vi "ex_HeaderToSprdsheetStr.vi"(6 "project":string, 7 "operator name":string, 8 "error in (no error)":errorcluster, 9 "Relative Time?":bool, 10 "file params in":T1={"delimiter"="\t", "origin time"=timestamp(0 s since 1904-01-01), "Flags"={"include col headings?"=TRUE, "x_columns"=0, "col headings always?"=TRUE, "time preference"=0, "hide col headings"=FALSE}, "Decimal Separator"=""} {"Flags"."time preference" items=["Absolute", "Relative"]; "Flags"."x_columns" items=["None", "One", "Multiple"]; "origin time" format="%<%X\n%x>T"}, 11 "description":string) -> (0 "error out":errorcluster, 1 "rows":i32, 2 "spreadsheet array":string[][](array[string]), 3 "spreadsheet string":string)   [LabVIEW 2020]
uses:
  <vilib>/express/express output/ExFileWriteBlock.llb/ex_WriteFileParams.ctl
  <vilib>/express/express input/ExFileReadBlock.llb/ex_ReadFileParams.ctl
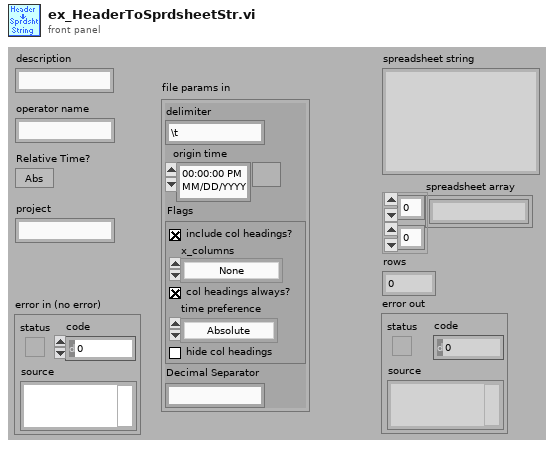
[diagram p1: front panel]
types:
  T1 = typedef "ex_WriteFileParams.ctl" = cluster{"delimiter":string, "origin time":timestamp, "Flags":T2, "Decimal Separator":string}
  T2 = typedef "ex_ReadFileParams.ctl" = cluster{"include col headings?":bool, "x_columns":u16, "col headings always?":bool, "time preference":u16, "hide col headings":bool}
  T3 = typedef "ex_SoftwareRevision.ctl" = cluster{"Major Version":u16, "Minor Version":u16}
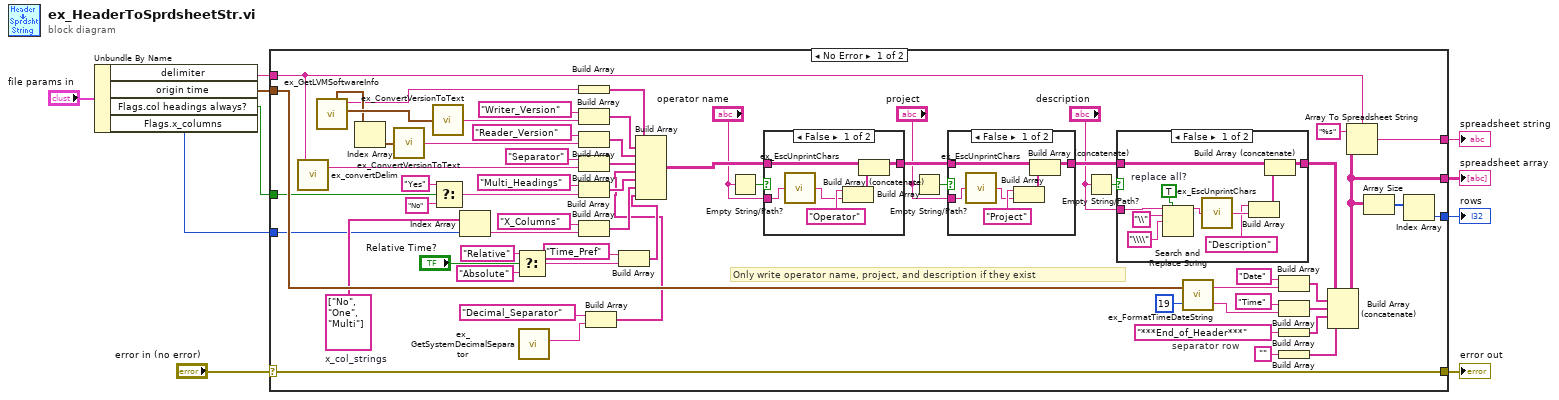
[diagram p0: block diagram]
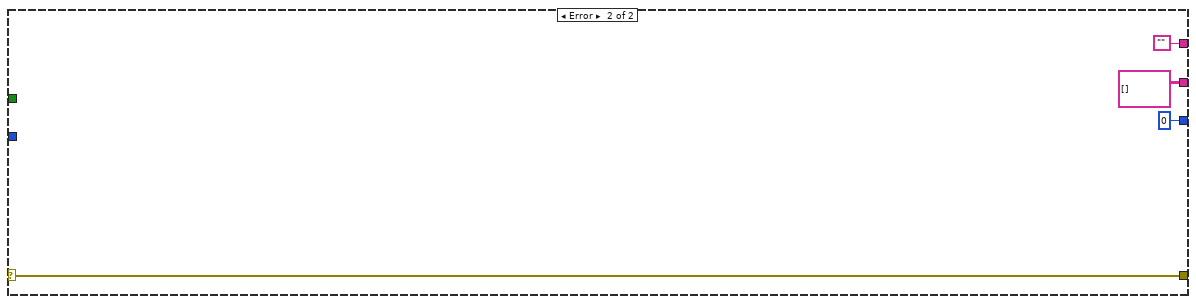
[diagram p5: hidden frame]
diagram:
  n1 = Unbundle By Name("file params in") -> ("delimiter"=w7:string, "origin time"=w6:timestamp, "Flags.col headings always?"=w5:bool, "Flags.x_columns"=w4:u16)
  n2 = case shown="No Error" "error in (no error)" {
    selector: "error in (no error)" -> [w63 w102]
    tunnel: [w63 w102] -> w9
    tunnel: w7 -> [w50 _]
    tunnel: w6 -> [w58 _]
    tunnel: w5 -> [w57 _]
    tunnel: w4 -> [w41 _]
    tunnel: [w20 ""] -> w3
    tunnel: [w19 string[][] []] -> w2
    tunnel: [w18 0] -> w1
    frame No Error {
      w42 = string[] ["No", "One", "Multi"]  # x_col_strings
      # "Only write operator name, project, and description if they exist"
      # "separator row"
      n3 = call <vilib>:"ex_convertDelim.vi"("delimiter in"=w50) -> ("delimiter out"=w51:string)  [unwired: 1 in, 1 out]
      n4 = call <vilib>:"ex_GetLVMSoftwareInfo.vi"() -> ("Version"=w39:T3, "Title"=w34:string, "Write Capabilities"=w37:T3[])  [unwired: 9 out]
      n5 = Index Array(array=w37) -> (element=w35:T3)  [unwired: 1 in]
      n6 = call <vilib>:"ex_ConvertVersionToText.vi"("Version"=w35) -> ("Text Version"=w36:string)
      n7 = call <vilib>:"ex_ConvertVersionToText.vi"("Version"=w39) -> ("Text Version"=w38:string)
      n8 = Select(t="Yes" ("hdr_str_yes"), s=w57, f="No" ("hdr_str_no")) -> (s? t:f=w67:string)
      n9 = Index Array(array=w42, index=w41) -> (element=w40:string)
      n10 = Select(t="Relative" ("hdr_str_yes"), s="Relative Time?", f="Absolute" ("hdr_str_yes")) -> (s? t:f=w49:string)
      n11 = call <vilib>:"ex_GetSystemDecimalSeparator.vi"() -> ("Decimal Seperator"=w11:string)  [unwired: 11 out]
      n12 = Build Array(w34) -> (w56:string[])
      n13 = Build Array("Writer_Version" ("element"), w38) -> (w53:string[])
      n14 = Build Array("Reader_Version" ("element"), w36) -> (w52:string[])
      n15 = Build Array("Separator", w51) -> (w72:string[])
      n16 = Build Array("Multi_Headings" ("hdr_str_rptcolhdgs"), w67) -> (w14:string[])
      n17 = Build Array("X_Columns" ("hdr_str_multtimecol"), w40) -> (w15:string[])
      n18 = Build Array("Decimal_Separator", w11) -> (w12:string[])
      n19 = Build Array("Time_Pref" ("hdr_str_rptcolhdgs"), w49) -> (w16:string[])
      n20 = Build Array(w56, w53, w52, w72, w12, w14, w15, w16) -> (w62:string[][])
      n21 = Empty String/Path?(string/path="operator name") -> (empty?=w29:bool)
      n22 = case shown="False" w29 {
        tunnel: w62 -> [w97 w98]
        tunnel: "operator name" -> [w92 _]
        tunnel: [w95 w98] -> w26
        frame False {
          n23 = call <vilib>:"ex_EscUnprintChars.vi"("input"=w92) -> ("output"=w93:string)
          n24 = Build Array("Operator" ("element"), w93) -> (w94:string[])
          n25 = Build Array (concatenate)(w97, w94) -> (w95:string[][])
        }
        frame True {
        }
      }
      n26 = Empty String/Path?(string/path="project") -> (empty?=w27:bool)
      n27 = case shown="False" w27 {
        tunnel: w26 -> [w90 w91]
        tunnel: "project" -> [w86 _]
        tunnel: [w88 w91] -> w23
        frame False {
          n28 = call <vilib>:"ex_EscUnprintChars.vi"("input"=w86) -> ("output"=w85:string)
          n29 = Build Array("Project" ("element"), w85) -> (w87:string[])
          n30 = Build Array (concatenate)(w90, w87) -> (w88:string[][])
        }
        frame True {
        }
      }
      n31 = Empty String/Path?(string/path="description") -> (empty?=w24:bool)
      n32 = case shown="False" w24 {
        tunnel: w23 -> [w83 w84]
        tunnel: "description" -> [w74 _]
        tunnel: [w82 w84] -> w21
        frame False {
          w79 = TRUE  # replace all?
          n33 = Search and Replace String(replace all?=w79, input string=w74, search string="\\" ("regular expression"), replace string="\\\\") -> (result string=w80:string)  [unwired: 1 in, 6 out]
          n34 = call <vilib>:"ex_EscUnprintChars.vi"("input"=w80) -> ("output"=w77:string)
          n35 = Build Array("Description" ("hdr_str_descr"), w77) -> (w75:string[])
          n36 = Build Array (concatenate)(w83, w75) -> (w82:string[][])
        }
        frame True {
        }
      }
      n37 = call <vilib>:"ex_FormatTimeDateString.vi"("seconds precision (3)"=u32 19, "seconds since 1/1/1904"=w58) -> ("time string"=w65:string, "date string"=w66:string)
      n38 = Build Array("Date" ("hdr_str_date"), w66) -> (w30:string[])
      n39 = Build Array("Time" ("hdr_str_time"), w65) -> (w31:string[])
      n40 = Build Array("***End_of_Header***" ("hdr_str_eoh")) -> (w32:string[])
      n41 = Build Array("" ("Empty String Constant")) -> (w33:string[])
      n42 = Build Array (concatenate)(w21, w30, w31, w32, w33) -> (w19:string[][])
      n43 = Array To Spreadsheet String(delimiter (Tab)=w50, array=w19, 3:"%s" ("format string")) -> (spreadsheet string=w20:string)
      n44 = Array Size(array=w19) -> (size(s)=w61:i32[])
      n45 = Index Array(array=w61) -> (element=w18:i32)  [unwired: 1 in]
    }
    frame Error {
    }
  }
  "error out" <- w9
  "rows" <- w1
  "spreadsheet array" <- w2
  "spreadsheet string" <- w3
